vi "SetPin.vi"(7 "Invert":bool, 8 "error in (no error)":errorcluster, 9 "Val":u16, 10 "Led num":u8, 11 "PCA in":refnum<class "PCA.lvclass">) -> (0 "error out":errorcluster, 3 "PCA out":refnum<class "PCA.lvclass">)   [LabVIEW 2022 SP3, in "PCA9685.lvlib" / "PCA.lvclass"]
uses:
  PCA.lvclass
  PCA.lvclass/PCA.ctl
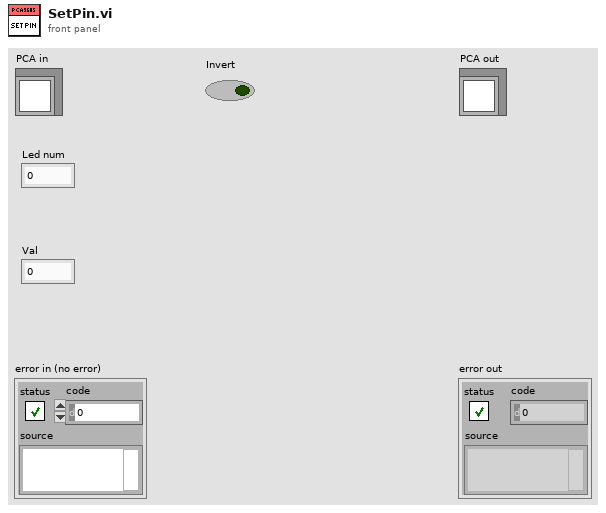
[diagram p1: front panel]
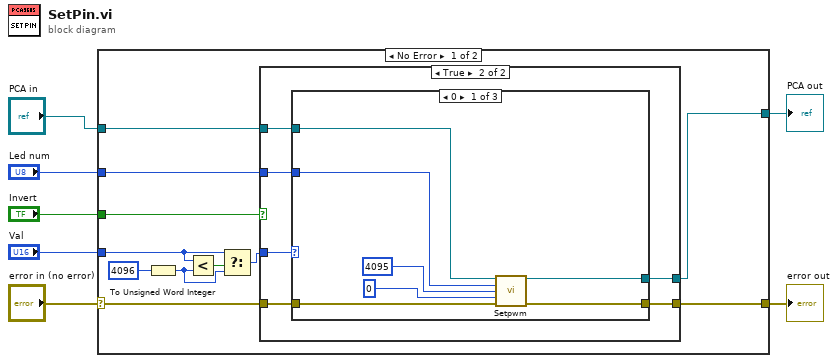
[diagram p0: block diagram]
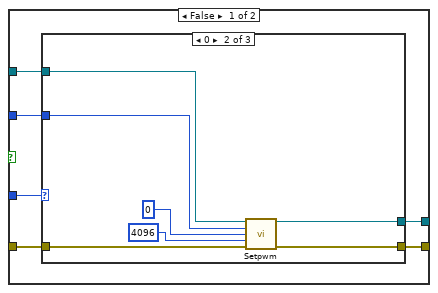
[diagram p2: hidden frame]
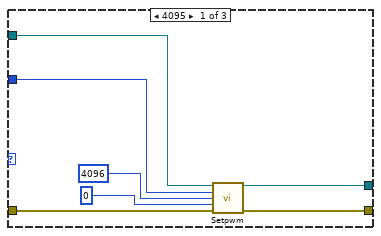
[diagram p3: hidden frame]
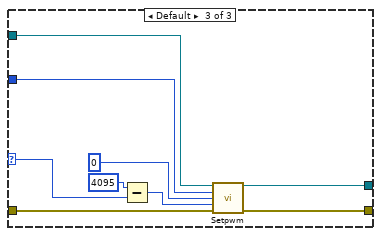
[diagram p4: hidden frame]
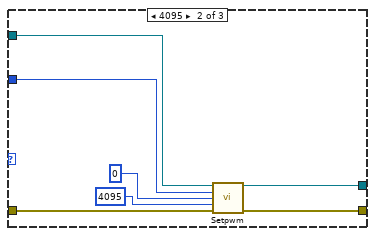
[diagram p5: hidden frame]
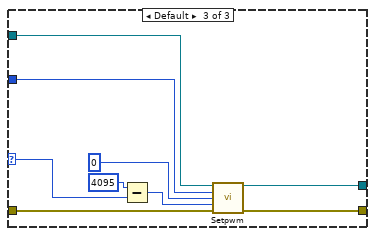
[diagram p6: hidden frame]
diagram:
  n1 = case shown="No Error" "error in (no error)" {
    selector: "error in (no error)" -> [w17 w78]
    tunnel: [w16 w78] -> w6
    tunnel: [w14 w77] -> w4
    tunnel: "PCA in" -> [w15 w77]
    tunnel: "Invert" -> [w18 _]
    tunnel: "Val" -> [w12 _]
    tunnel: "Led num" -> [w13 _]
    frame No Error {
      n2 = To Unsigned Word Integer(number=4096) -> (unsigned 16bit integer=w9:u16)
      n3 = Less?(x=w12, y=w9) -> (x < y?=w11:bool)
      n4 = Select(t=w12, s=w11, f=w9) -> (s? t:f=w8:u16)
      n5 = case shown="True" w18 {
        tunnel: w8 -> [w23 w53]
        tunnel: w17 -> [w24 w52]
        tunnel: [w19 w51] -> w16
        tunnel: w15 -> [w21 w50]
        tunnel: [w20 w49] -> w14
        tunnel: w13 -> [w22 w48]
        frame False {
          n6 = case shown="0" w23 {
            selector: w23 -> [_ _ w41]
            tunnel: w24 -> [w31 w38 w47]
            tunnel: [w30 w37 w46] -> w19
            tunnel: w21 -> [w29 w36 w45]
            tunnel: [w28 w35 w44] -> w20
            tunnel: w22 -> [w27 w33 w43]
            frame 4095 {
              n7 = call "Setpwm.vi"("PCA in"=w29, "Led num"=w27, "on"=4096, "off"=0, "error in (no error)"=w31) -> ("PCA out"=w28:refnum<class "PCA.lvclass">, "error out"=w30:errorcluster)  [unwired: 8 in, 1 out]
            }
            frame 0 {
              n8 = call "Setpwm.vi"("PCA in"=w36, "Led num"=w33, "on"=0, "off"=4096, "error in (no error)"=w38) -> ("PCA out"=w35:refnum<class "PCA.lvclass">, "error out"=w37:errorcluster)  [unwired: 8 in, 1 out]
            }
            frame Default {
              n9 = Subtract(x=4095, y=w41) -> (x-y=w39:i32)
              n10 = call "Setpwm.vi"("PCA in"=w45, "Led num"=w43, "on"=0, "off"=w39, "error in (no error)"=w47) -> ("PCA out"=w44:refnum<class "PCA.lvclass">, "error out"=w46:errorcluster)  [unwired: 8 in, 1 out]
            }
          }
        }
        frame True {
          n11 = case shown="0" w53 {
            selector: w53 -> [_ _ w70]
            tunnel: w52 -> [w60 w67 w76]
            tunnel: [w59 w66 w75] -> w51
            tunnel: w50 -> [w58 w65 w74]
            tunnel: [w57 w64 w73] -> w49
            tunnel: w48 -> [w56 w62 w72]
            frame 0 {
              n12 = call "Setpwm.vi"("PCA in"=w58, "Led num"=w56, "on"=4095, "off"=0, "error in (no error)"=w60) -> ("PCA out"=w57:refnum<class "PCA.lvclass">, "error out"=w59:errorcluster)  [unwired: 8 in, 1 out]
            }
            frame 4095 {
              n13 = call "Setpwm.vi"("PCA in"=w65, "Led num"=w62, "on"=0, "off"=4095, "error in (no error)"=w67) -> ("PCA out"=w64:refnum<class "PCA.lvclass">, "error out"=w66:errorcluster)  [unwired: 8 in, 1 out]
            }
            frame Default {
              n14 = Subtract(x=4095, y=w70) -> (x-y=w68:i32)
              n15 = call "Setpwm.vi"("PCA in"=w74, "Led num"=w72, "on"=0, "off"=w68, "error in (no error)"=w76) -> ("PCA out"=w73:refnum<class "PCA.lvclass">, "error out"=w75:errorcluster)  [unwired: 8 in, 1 out]
            }
          }
        }
      }
    }
    frame Error {
    }
  }
  "error out" <- w6
  "PCA out" <- w4
